vi "1. Color Class and Pattern Match.vi"() -> ()   [LabVIEW 2019]
doc: "c 2020 ReMiSYS All rights reserved."
panel:
  out "Classes (Color Classification 1) 2":string[](array[string])
  out "Image Out 2":T1(plugin-control)
  out "Classes (Color Classification 1)":string[](array[string])
  out "Array 2":enum16{"Cross", "Tringle", "Square", "Hex"}[](array[ring])
  out "Array":enum16{"Cross", "Tringle", "Square", "Hex"}[](array[ring])
  in  "Stop Button":bool
  out "Image Out":T1(plugin-control)
  # "c 2021 ReMiSYS All rights reserved."
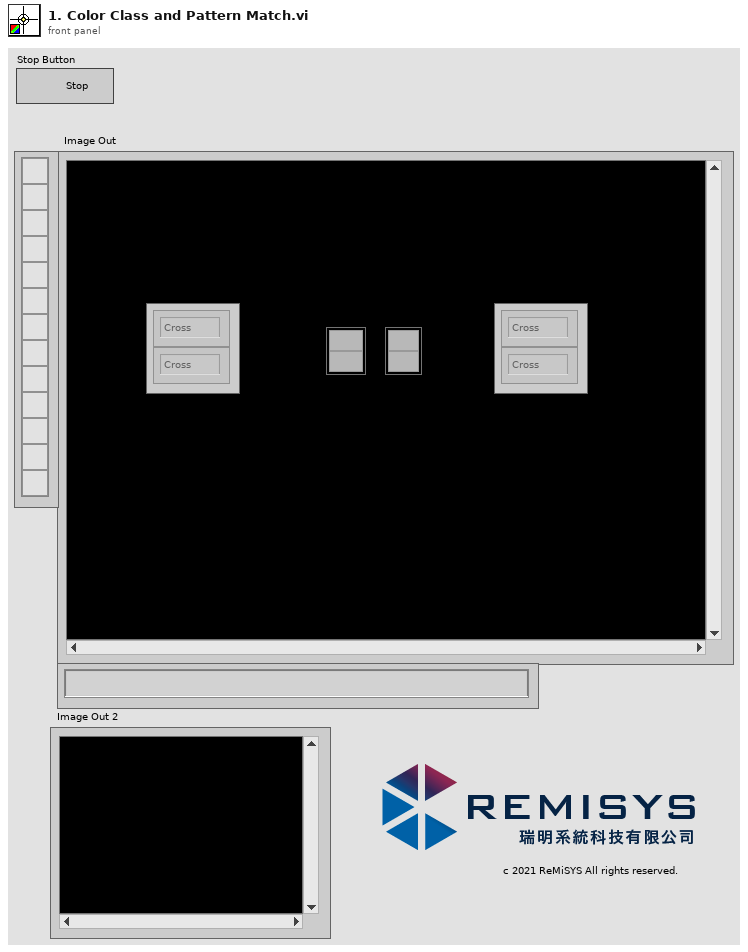
[diagram p1: front panel]
types:
  T1 = typedef "IMAQ Image.ctl" = refnum<image>
  T2 = typedef "Image Type" = u32
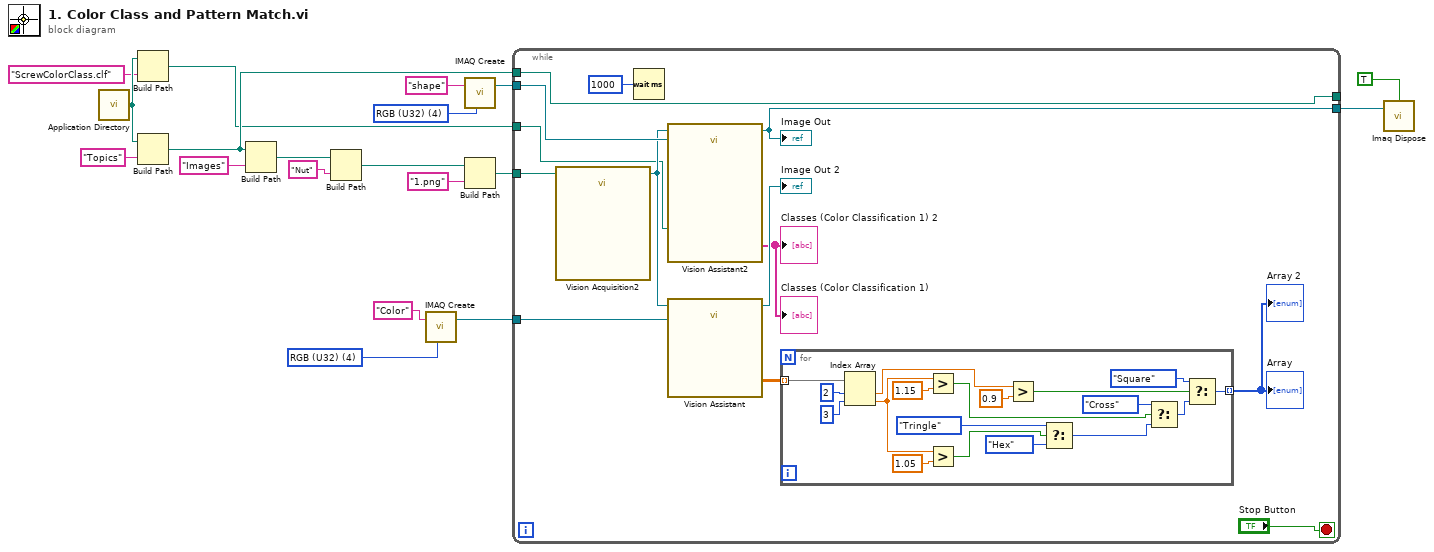
[diagram p0: block diagram]
diagram:
  w6 = T2 4 items=["Grayscale (U8)", "Grayscale (I16)", "Grayscale (SGL)", "Complex (CSG)", "RGB (U32)", "HSL (U32)", "RGB (U64)", "Grayscale (U16)"] ("Image Type")
  w15 = T2 4 items=["Grayscale (U8)", "Grayscale (I16)", "Grayscale (SGL)", "Complex (CSG)", "RGB (U32)", "HSL (U32)", "RGB (U64)", "Grayscale (U16)"] ("Image Type")
  n1 = call <vilib>:"Application Directory.vi"() -> ("Application Directory"=w3:path)
  n2 = Build Path(base path=w3, name or relative path="ScrewColorClass.clf") -> (appended path=w1:path)
  n3 = Build Path(base path=w3, name or relative path="Topics") -> (appended path=w7:path)
  n4 = Build Path(base path=w7, name or relative path="Images") -> (appended path=w8:path)
  n5 = Build Path(base path=w8, name or relative path="Nut") -> (appended path=w10:path)
  n6 = call "IMAQ Create"("Image Name"="Color", "Image Type"=w6) -> ("New Image"=w4:T1)  [unwired: 3 in, 1 out]
  n7 = call "IMAQ Create"("Image Name"="shape", "Image Type"=w15) -> ("New Image"=w16:T1)  [unwired: 3 in, 1 out]
  n8 = Build Path(base path=w10, name or relative path="1.png") -> (appended path=w9:path)
  n9 = while {
    tunnel: [w24] -> w18
    tunnel: w16 -> [w32]
    tunnel: w9 -> [w31]
    tunnel: [w30] -> _
    tunnel: w7 -> [w30]
    tunnel: w4 -> [w23]
    tunnel: w1 -> [w20]
    stop <- "Stop Button" stop-if-true
    n10 = call "Vision Acquisition2"("Image Path"=w31) -> ("Image Out"=w22:T1)  [unwired: 2 in, 24 out]
    n11 = Wait (ms)(milliseconds to wait=u32 1000) -> ()  [unwired: 1 out]
    n12 = call "Vision Assistant2"("Image In"=w22, "Image Dst"=w32, "File Path (Color Classification 1)"=w20) -> ("Image Out"=w24:T1, "Classes (Color Classification 1)"=→"Classes (Color Classification 1)" →"Classes (Color Classification 1) 2":string[])  [unwired: 22 in, 1 out]
    "Image Out" <- w24
    n13 = call "Vision Assistant"("Image In"=w22, "Image Dst"=w23) -> ("Image Out"=→"Image Out 2":T1, "Particle Measurements (Pixels) (Particle Analysis 1)"=w27:dbl[][])  [unwired: 22 in, 2 out]
    n14 = for {
      tunnel: w27 -> [w50] mode=indexing
      tunnel: [w35] -> w26 mode=indexing
      n15 = Index Array(array=w50, index #1=2 ("index"), index #2=3 ("index")) -> (element #1=w49:dbl, element #2=w46:dbl)
      n16 = Greater?(x=w46, y=1.15) -> (0:w38:bool)
      n17 = Greater?(x=w46, y=1.05) -> (0:w45:bool)
      n18 = Greater?(x=w49, y=0.9) -> (0:w40:bool)
      n19 = Select(t=enum16{"Cross", "Tringle", "Square", "Hex"}."Tringle", s=w45, f=enum16{"Cross", "Tringle", "Square", "Hex"}."Hex") -> (s? t:f=w42:enum16{"Cross", "Tringle", "Square", "Hex"})
      n20 = Select(t=enum16{"Cross", "Tringle", "Square", "Hex"}."Cross", s=w38, f=w42) -> (s? t:f=w41:enum16{"Cross", "Tringle", "Square", "Hex"})
      n21 = Select(t=enum16{"Cross", "Tringle", "Square", "Hex"}."Square", s=w40, f=w41) -> (s? t:f=w35:enum16{"Cross", "Tringle", "Square", "Hex"})
    }
    "Array 2" <- w26
    "Array" <- w26
  }
  n22 = call "Imaq Dispose"("All Images? (No)"=TRUE, "Image"=w18) -> ()  [unwired: 4 in, 1 out]
